vi "Get voltage and currents.vi"(0 "Zaber":T1={"Serial port handle"="", "Axis"="", "Controller #"=0, "Min position"=0.0, "Max position"=0.0, "Min velocity"=0.0, "Max velocity"=0.0, "Firmware"="", "Device ID"=0, "Variable event"=refnum, "Variable ref"=refnum, "Resolution, usteps/step"=0, "Serial port semaphore"=refnum, "Joystick buttons"={"MinDir"=1, "MaxDir"=2, "MedSpeed"=5, "HighSpeed"=6}} {"Joystick buttons"."HighSpeed" min=1 max=25 step=1; "Joystick buttons"."MedSpeed" min=1 max=25 step=1; "Joystick buttons"."MaxDir" min=1 max=25 step=1; "Joystick buttons"."MinDir" min=1 max=25 step=1}, 5 "error in":errorcluster) -> (14 "Zaber out":T1={"Serial port handle"="", "Axis"="", "Controller #"=0, "Min position"=0.0, "Max position"=0.0, "Min velocity"=0.0, "Max velocity"=0.0, "Firmware"="", "Device ID"=0, "Variable event"=refnum, "Variable ref"=refnum, "Resolution, usteps/step"=0, "Serial port semaphore"=refnum, "Joystick buttons"={"MinDir"=1, "MaxDir"=2, "MedSpeed"=5, "HighSpeed"=6}} {"Joystick buttons"."HighSpeed" min=1 max=25 step=1; "Joystick buttons"."MedSpeed" min=1 max=25 step=1; "Joystick buttons"."MaxDir" min=1 max=25 step=1; "Joystick buttons"."MinDir" min=1 max=25 step=1}, 15 "Voltage, V":dbl, 17 "Running current, mA":dbl, 18 "Holding current, mA":dbl, 19 "error out":errorcluster)   [LabVIEW 2017]
uses:
  CommandZaber.ctl
  GenericDataEvent/GenericEvent.ctl
  Zaber.ctl
  ZaberVariables.ctl
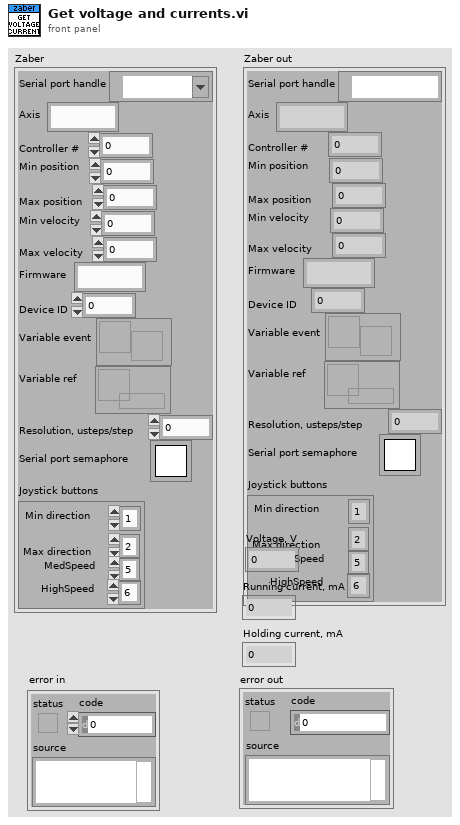
[diagram p1: front panel]
types:
  T1 = typedef "Zaber.ctl" = cluster{"Serial port handle":refnum<visa-resource-name>, "Axis":string, "Controller #":u8, "Min position":dbl, "Max position":dbl, "Min velocity":dbl, "Max velocity":dbl, "Firmware":string, "Device ID":i32, "Variable event":T2, "Variable ref":refnum<data-value>, "Resolution, usteps/step":i32, "Serial port semaphore":T3, "Joystick buttons":cluster{"MinDir":i32, "MaxDir":i32, "MedSpeed":i32, "HighSpeed":i32}}
  T2 = typedef "GenericEvent.ctl" = refnum<user-event>
  T3 = typedef "Semaphore RefNum" = refnum<k1>
  T4 = typedef "CommandZaber.ctl" = cluster{"Command":u8, "Data":i32}
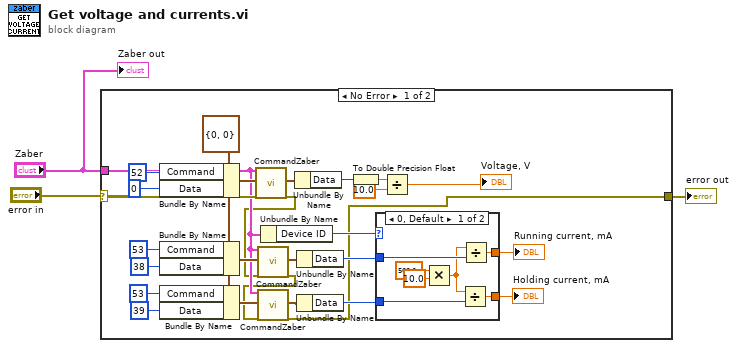
[diagram p0: block diagram]
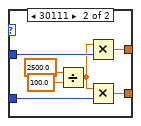
[diagram p2: hidden frame]
diagram:
  n1 = case shown="No Error" "error in" {
    selector: "error in" -> [w13 w45]
    tunnel: [w4 w45] -> w1
    tunnel: "Zaber" -> [w12 _]
    frame No Error {
      w14 = T4 {"Command"=0, "Data"=0} ("Command")
      n2 = Bundle By Name(cluster=w14, "Command"=52 ("Data"), "Data"=0) -> (w28:T4)
      n3 = Bundle By Name(cluster=w14, "Command"=53 ("Data"), "Data"=38) -> (w21:T4)
      n4 = Bundle By Name(cluster=w14, "Command"=53 ("Data"), "Data"=39) -> (w15:T4)
      n5 = call "CommandZaber.vi"("Zaber"=w12, "Command"=w28, "error in"=w13) -> ("Answer"=w27:T4, "error out"=w5:errorcluster)  [unwired: 13 in, 2 out]
      n6 = call "CommandZaber.vi"("Zaber"=w12, "Command"=w21, "error in"=w5) -> ("Answer"=w22:T4, "error out"=w6:errorcluster)  [unwired: 13 in, 2 out]
      n7 = call "CommandZaber.vi"("Zaber"=w12, "Command"=w15, "error in"=w6) -> ("Answer"=w18:T4, "error out"=w4:errorcluster)  [unwired: 13 in, 2 out]
      n8 = Unbundle By Name(w12) -> ("Device ID"=w11:i32)
      n9 = Unbundle By Name(w27) -> ("Data"=w26:i32)
      n10 = Unbundle By Name(w22) -> ("Data"=w10:i32)
      n11 = Unbundle By Name(w18) -> ("Data"=w9:i32)
      n12 = To Double Precision Float(number=w26) -> (double precision float=w25:dbl)
      n13 = case shown="0, Default" w11 {
        tunnel: [w35 w43] -> w8
        tunnel: w10 -> [w34 w42]
        tunnel: w9 -> [w32 w41]
        tunnel: [w31 w40] -> w7
        frame 0, Default {
          n14 = Multiply(x=500.0, y=10.0) -> (x*y=w33:dbl)
          n15 = Divide(x=w33, y=w32) -> (x/y=w31:dbl)
          n16 = Divide(x=w33, y=w34) -> (x/y=w35:dbl)
        }
        frame 30111 {
          n17 = Divide(x=2500.0, y=100.0) -> (x/y=w38:dbl)
          n18 = Multiply(x=w38, y=w42) -> (x*y=w43:dbl)
          n19 = Multiply(x=w38, y=w41) -> (x*y=w40:dbl)
        }
      }
      "Running current, mA" <- w8
      "Holding current, mA" <- w7
      n20 = Divide(x=w25, y=10.0) -> (x/y=→"Voltage, V":dbl)
    }
    frame Error {
    }
  }
  "error out" <- w1
  "Zaber out" <- "Zaber"
